vi "CommunicatorManager.vi"(8 "error in (no error)":errorcluster, 11 "TCPCommunicator in":refnum<class "TCPCommunicator.lvclass">) -> (0 "error out":errorcluster, 3 "TCPCommunicator out":refnum<class "TCPCommunicator.lvclass">)   [LabVIEW 2016, in "TCPCommunicator.lvclass"]
uses:
  TCPCommunicator.lvclass
panel:
  out "String":string
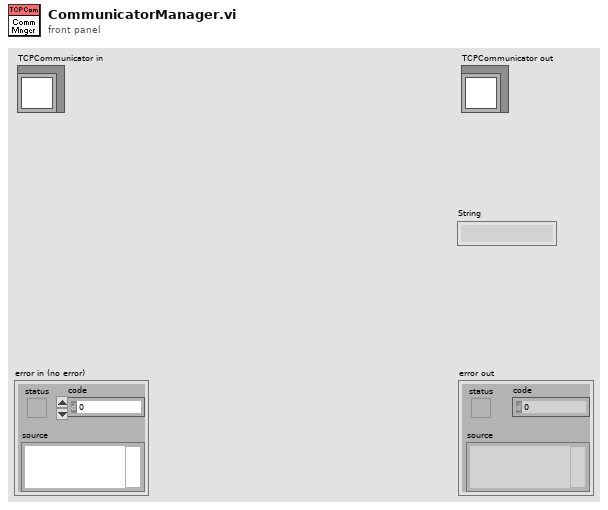
[diagram p1: front panel]
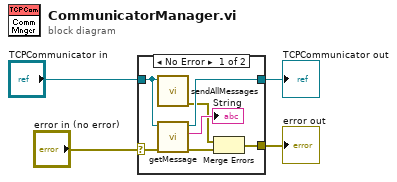
[diagram p0: block diagram]
diagram:
  n1 = case shown="No Error" "error in (no error)" {
    selector: "error in (no error)" -> [w10 w13]
    tunnel: [w9 w13] -> w1
    tunnel: [w11 w12] -> w3
    tunnel: "TCPCommunicator in" -> [w5 w12]
    frame No Error {
      n2 = call-dynamic "sendAllMessages.vi"("TCPCommunicator in"=w5) -> ("error out"=w6:errorcluster)  [unwired: 9 in, 1 out]
      n3 = call-dynamic "getMessage.vi"("error in (no error)"=w10, "TCPCommunicator in"=w5) -> ("error out"=w8:errorcluster, "String"=→"String":string, "TCPCommunicator out"=w11:refnum<class "TCPCommunicator.lvclass">)  [unwired: 7 in]
      n4 = Merge Errors(w6, w8) -> (w9:errorcluster)
    }
    frame Error {
    }
  }
  "error out" <- w1
  "TCPCommunicator out" <- w3
